vi "TTA_MATLAB_RFIC_Perform1TilePALTest.vi"(0 "Channel":string(combo), 1 "MXG VISA Resource In":refnum<visa-resource-name>, 2 "EXA VISA Resource":refnum<visa-resource-name>, 5 "Tx":string(combo), 7 "Freq_Cal_List":dbl[](array[numeric]), 11 "error in":errorcluster) -> (12 "MXG VISA Resource Out":refnum<visa-resource-name>, 13 "EXA VISA Resource Out":refnum<visa-resource-name>, 15 "error out":errorcluster)   [LabVIEW 2016]
uses:
  TTA_Globals/TTA_Global_Complete_Settings.vi
panel:
  out "IF Index":i32
  in  "PALLinearization Values":T1
  out "Tx#":i32
  out "CH#":i32
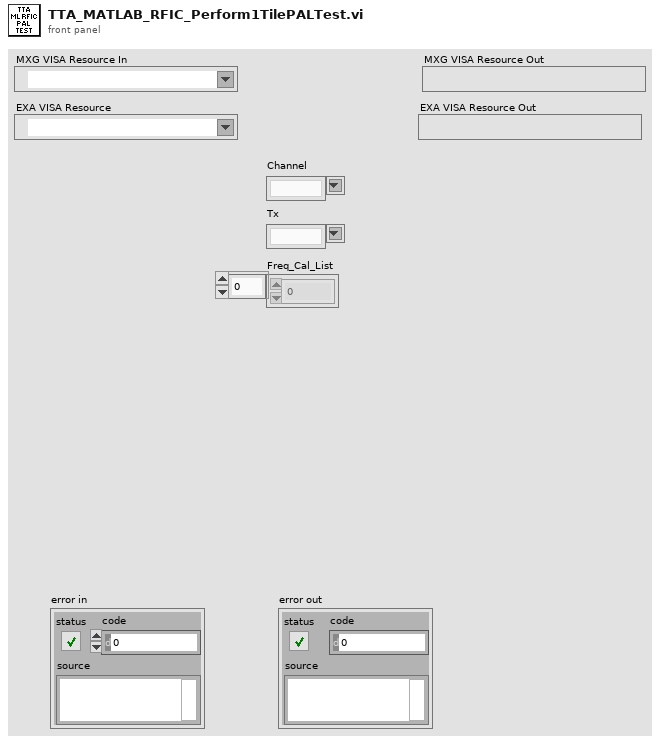
[diagram p1: front panel]
types:
  T1 = cluster{"Tx IF Offsets":dbl[], "ACPR Filename":string, "Sampling Rate":dbl, "TxIF_Freq":dbl, "Power (dBm)":dbl, "IF Frequency Sweep (MHz)":dbl[], "BDSFreq":dbl, "Amplitude Range\nMax(dBm)":dbl, "Amplitude Range\nMin(dBm)":dbl, "CAL Amplitude\nIncrement(dB)":dbl, "CAL Amplitude\nDecrement (dB)":dbl, "Amplitude Least\nCriteria (dBm)":dbl}
  T2 = typedef "TTA_Control_Complete_Settings_Cluster.ctl" = cluster{"Brief Cluster":cluster{"STM Firmware File":string, "STM Firmware Address":string, "Required SW Version":string, "Template Used":string}, "Instrument Setting Cluster":cluster{"BDSFreq":dbl, "BDS Amp":dbl, "TxRFCal_Freq":dbl, "TxRFCal_Amp":dbl, "RxRFCal_Freq":dbl, "RxRFCal_Freq":dbl, "TxIF_Freq":dbl, "TxIF_Amp":dbl, "Tx_Output_Power_Signal_Freq":dbl, "Tx_ACPR_Signal_Freq":dbl, "Rx_RF_Freq":dbl, "Rx_RF_Amp":dbl, "Rx_Output_Power_Signal_Freq":dbl, "Rx_Output_Power_Sense_Freq":dbl}, "PAL Calibration\nInputs Cluster":cluster{"Amplitude Range\nMax(dBm)":dbl, "Amplitude Range\nMin(dBm)":dbl, "Amplitude Least\nCriteria (dBm)":dbl, "Frequency 1":dbl, "Frequency 2":dbl, "Frequency 3":dbl, "CAL Amplitude\nDecrement (dB)":dbl, "CAL Amplitude\nIncrement(dB)":dbl, "DownloadFile":string}, "TxOffset Cal Cluster":cluster{"Tx1 Offset (dB)":dbl, "Tx2 Offset (dB)":dbl, "Tx3 Offset (dB)":dbl, "Tx4 Offset (dB)":dbl, "Total RF Tx Loss (dB)":dbl}, "RxOffset Cal Cluster":cluster{"Rx1 Offset (dB)":dbl, "Rx2 Offset (dB)":dbl, "Rx3 Offset (dB)":dbl, "Rx4 Offset (dB)":dbl, "Total RF Rx Loss (dB)":dbl}, "TX Output Power Settings Cluster":cluster{"Frequency Sweep (MHz)":dbl[], "Sig Gen \nPower (dBm)":dbl, "Span (kHz)":dbl, "RBW (Hz)":dbl, "Ref Level (dBm)":dbl, "Low Power \nLimit":dbl, "High Power \nLimit":dbl, "DigAtt Max":dbl, "DigAtt Min":dbl}, "Tx ACPR Settings Cluster":cluster{"ACPR Filename":string, "Sampling Rate":dbl, "Power (dBm)":dbl, "IF Frequency Sweep (MHz)":dbl[], "State Name":string, "Mechanical\nAttenuation":dbl, "RefLevel Offset":dbl, "Amplitude Range\nMax (dBm)":dbl, "Amplitude Range\nMin (dBm)":dbl, "Cal Amp \nIncrement (dB)":dbl, "Cal Amp\nDecrement (dB)":dbl}, "Power Cal Cluster":cluster{"Power List (dBm)":dbl[], "Frequency (MHz)":dbl[], "Cal Decrement (dB)":dbl, "Cal Increment (dB)":dbl}, "Rx Received Power Settings Cluster":cluster{"Frequency Sweep (MHz)":dbl[], "Power (dBm)":dbl, "Span (kHz)":dbl, "RBW (Hz)":dbl, "Ref Level":dbl, "Low Power \nLimit (dBm)":dbl, "High Power\nLimit (dBm)":dbl}, "Tx Output Power Criteria Cluster":cluster{"CH1-TX1 \nMin":dbl, "CH1-TX1\nMax":dbl, "CH1-TXx3\nMin ":dbl, "CH1-TXx3\nMax":dbl, "CH2-TX1\nMin":dbl, "CH2-TX1\nMax":dbl, "CH2-TXx3\nMin":dbl, "CH2-TXx3\nMax":dbl}, "Tx ACPR Criteria Cluster":cluster{"Min Inband":dbl, "Max Close Outband":dbl, "Max Far Outband":dbl}, "Rx Output Power Criteria Cluster":cluster{"CH1-RX1 \nMin":dbl, "CH1-RX1 \nMax":dbl, "CH1-RXx3 \nMin":dbl, "CH1-RXx3\nMax":dbl, "CH2-RX1\nMin":dbl, "CH2-RX1\nMax":dbl, "CH2-RXx3\nMin":dbl, "CH2-RXx3\nMax":dbl}}
  T3 = cluster{"BDSFreq":dbl, "BDS Amp":dbl, "TxRFCal_Freq":dbl, "TxRFCal_Amp":dbl, "RxRFCal_Freq":dbl, "RxRFCal_Freq":dbl, "TxIF_Freq":dbl, "TxIF_Amp":dbl, "Tx_Output_Power_Signal_Freq":dbl, "Tx_ACPR_Signal_Freq":dbl, "Rx_RF_Freq":dbl, "Rx_RF_Amp":dbl, "Rx_Output_Power_Signal_Freq":dbl, "Rx_Output_Power_Sense_Freq":dbl}
  T4 = cluster{"Amplitude Range\nMax(dBm)":dbl, "Amplitude Range\nMin(dBm)":dbl, "Amplitude Least\nCriteria (dBm)":dbl, "Frequency 1":dbl, "Frequency 2":dbl, "Frequency 3":dbl, "CAL Amplitude\nDecrement (dB)":dbl, "CAL Amplitude\nIncrement(dB)":dbl, "DownloadFile":string}
  T5 = cluster{"Tx1 Offset (dB)":dbl, "Tx2 Offset (dB)":dbl, "Tx3 Offset (dB)":dbl, "Tx4 Offset (dB)":dbl, "Total RF Tx Loss (dB)":dbl}
  T6 = cluster{"ACPR Filename":string, "Sampling Rate":dbl, "Power (dBm)":dbl, "IF Frequency Sweep (MHz)":dbl[], "State Name":string, "Mechanical\nAttenuation":dbl, "RefLevel Offset":dbl, "Amplitude Range\nMax (dBm)":dbl, "Amplitude Range\nMin (dBm)":dbl, "Cal Amp \nIncrement (dB)":dbl, "Cal Amp\nDecrement (dB)":dbl}
  T7 = cluster{"Amplitude Range\nMax(dBm)":dbl, "Amplitude Range\nMin(dBm)":dbl, "CAL Amplitude\nDecrement (dB)":dbl, "CAL Amplitude\nIncrement(dB)":dbl, "Amplitude Least\nCriteria (dBm)":dbl}
  T8 = enum16{"TX1", "TX2", "TX3", "TX4", "TXx3", "TXx4", "RX1", "RX2", "RX3", "RX4", "RXx3", "RXx4", "RFCal"}
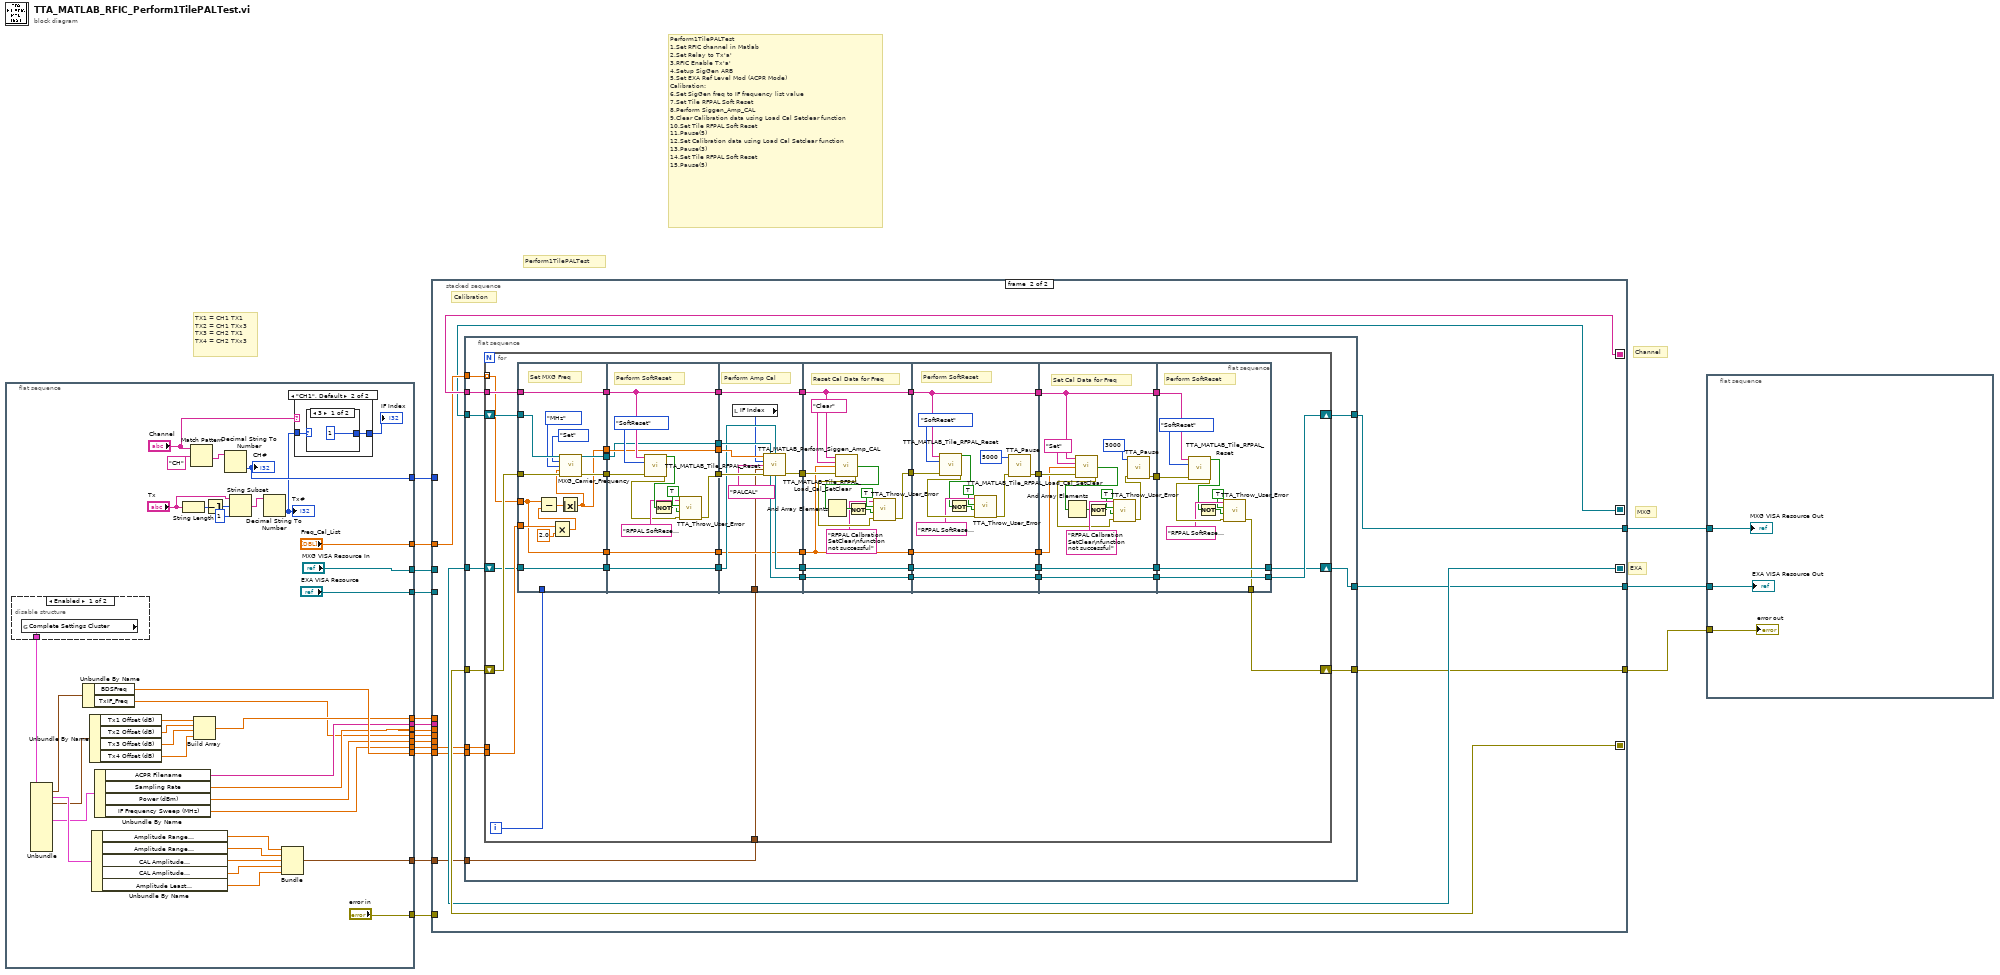
[diagram p0: block diagram]
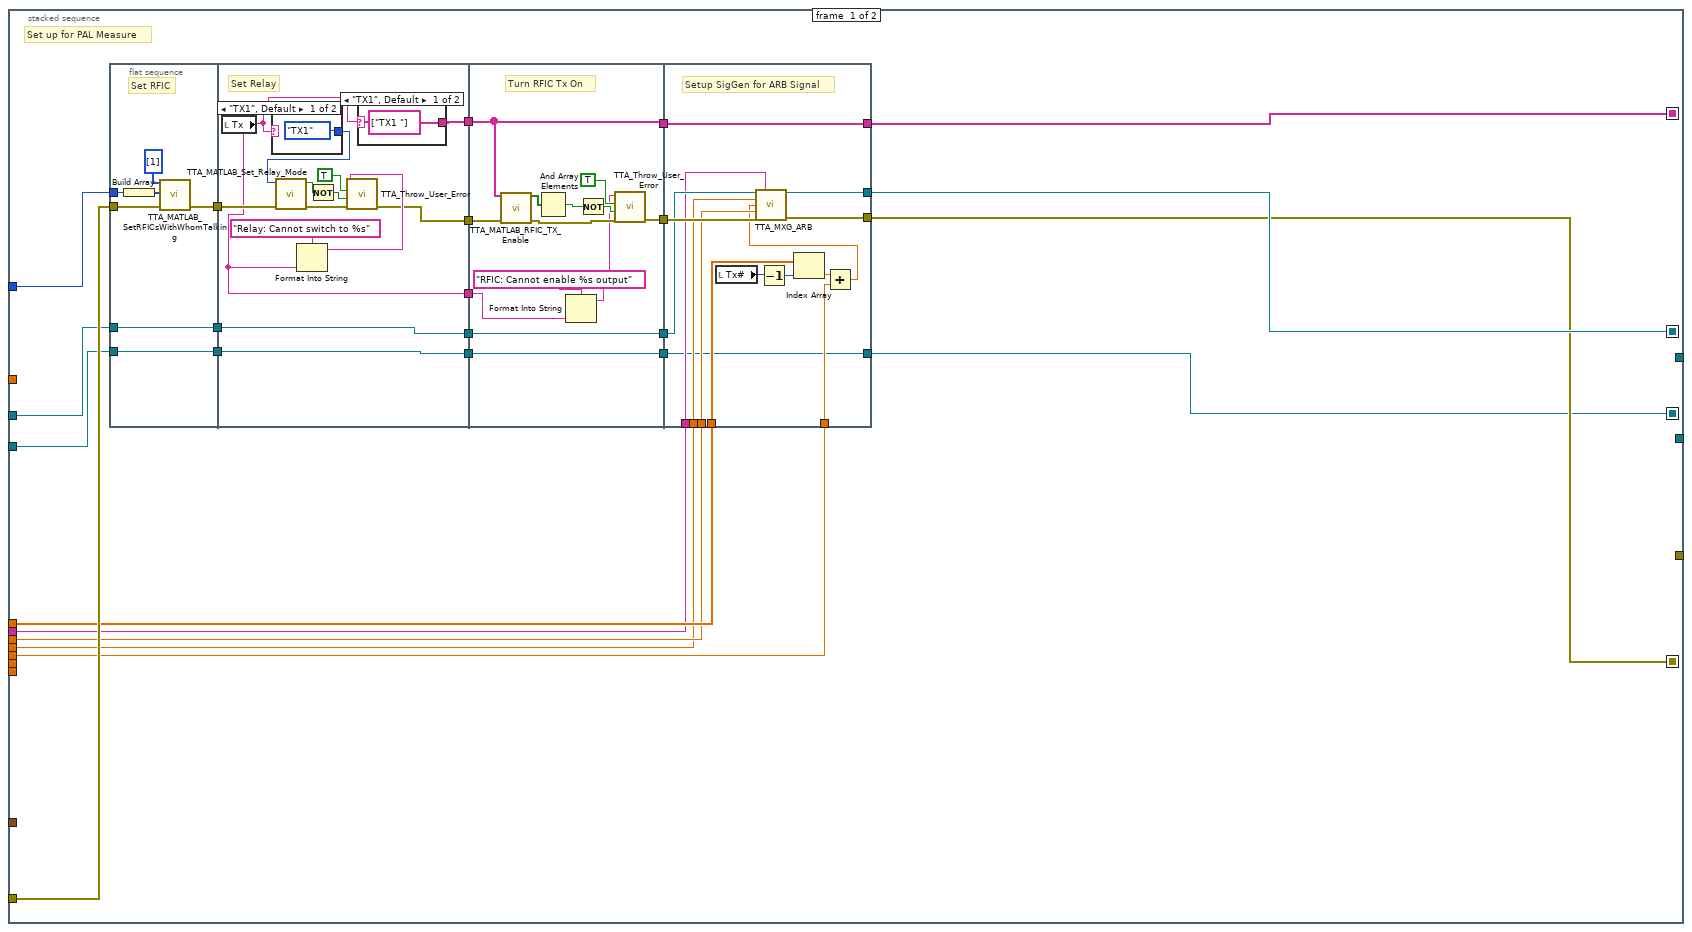
[diagram p2: hidden frame]
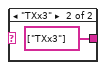
[diagram p3: hidden frame]
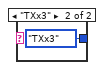
[diagram p4: hidden frame]
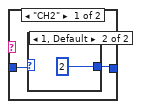
[diagram p5: hidden frame]
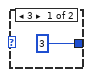
[diagram p6: hidden frame]
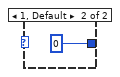
[diagram p7: hidden frame]
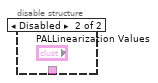
[diagram p8: hidden frame]
diagram:
  # "TX1 = CH1 TX1\nTX2 = CH1 TXx3\nTX3 = CH2 TX1\nTX4 = CH2 TXx3"
  # "Perform1TilePALTest\n1.Set RFIC channel in Matlab\n2.Set Relay to Tx'a'\n3.RFIC Enable Tx'a'\n4.Setup SigGen ARB\n5.Set EXA Ref Level Mod (ACPR Mode)\nCalibration:\n6.Set SigGen freq to IF frequency list value\n7.Set Tile RFPAL Soft Reset\n8.Perform Siggen_Amp_CAL \n9.Clear Calibration data using Load Cal Setclear function\n10.Set Tile RFPAL Soft Reset\n11.Pause(5)\n12.Set Calibration data using Load Cal Setclear function\n13.Pause(3)\n14.Set Tile RFPAL Soft Reset\n15.Pause(5)"
  # "EXA"
  # "MXG"
  # "Channel"
  # "Perform1TilePALTest"
  n1 = flat-sequence {
    tunnel: ["error in"] -> w16
    tunnel: ["MXG VISA Resource In"] -> w14
    tunnel: ["EXA VISA Resource"] -> w13
    tunnel: [w48] -> w15
    tunnel: ["Freq_Cal_List"] -> w10
    tunnel: [w27] -> w9
    tunnel: [w32] -> w8
    tunnel: [w30] -> w7
    tunnel: [w31] -> w6
    tunnel: [w29] -> w5
    tunnel: [w28] -> w4
    tunnel: [w37] -> w3
    tunnel: [w17] -> w2
    frame #0 {
      n2 = disable-structure shown="Enabled" {
        disable-tunnel: [w62 _] -> w42
        frame Enabled {
          n3 = global read "TTA_Global_Complete_Settings.vi" "Complete Settings Cluster"() -> (w62:T2)
        }
        frame Disabled {
        }
      }
      n4 = Unbundle(w42) -> ("Instrument Setting Cluster"=w41:T3, "PAL Calibration\nInputs Cluster"=w40:T4, "TxOffset Cal Cluster"=w39:T5, "Tx ACPR Settings Cluster"=w38:T6)  [unwired: 8 out]
      n5 = Unbundle By Name(w41) -> ("BDSFreq"=w37:dbl, "TxIF_Freq"=w27:dbl)
      n6 = Unbundle By Name(w39) -> ("Tx1 Offset (dB)"=w36:dbl, "Tx2 Offset (dB)"=w35:dbl, "Tx3 Offset (dB)"=w34:dbl, "Tx4 Offset (dB)"=w33:dbl)
      n7 = Unbundle By Name(w40) -> ("Amplitude Range\nMax(dBm)"=w22:dbl, "Amplitude Range\nMin(dBm)"=w21:dbl, "CAL Amplitude\nDecrement (dB)"=w20:dbl, "CAL Amplitude\nIncrement(dB)"=w19:dbl, "Amplitude Least\nCriteria (dBm)"=w18:dbl)
      n8 = Unbundle By Name(w38) -> ("ACPR Filename"=w31:string, "Sampling Rate"=w30:dbl, "Power (dBm)"=w29:dbl, "IF Frequency Sweep (MHz)"=w28:dbl[])
      n9 = String Length(string="Tx") -> (length=w47:i32)
      n10 = Match Pattern(string="Channel", regular expression="CH") -> (after substring=w49:string)  [unwired: 1 in, 3 out]
      n11 = Build Array(w36, w35, w34, w33) -> (w32:dbl[])
      n12 = Decrement(x=w47) -> (x-1=w46:i32)
      n13 = Decimal String To Number(string=w49) -> (number=w48:i32)  [unwired: 2 in, 1 out]
      "CH#" <- w48
      n14 = String Subset(string="Tx", offset (0)=w46, length (rest)=1 ("length (rest)")) -> (substring=w44:string)
      n15 = Decimal String To Number(string=w44) -> (number=w24:i32)  [unwired: 2 in, 1 out]
      "Tx#" <- w24
      n16 = Bundle("Amplitude Range\nMax(dBm)"=w22, "Amplitude Range\nMin(dBm)"=w21, "CAL Amplitude\nDecrement (dB)"=w20, "CAL Amplitude\nIncrement(dB)"=w19, "Amplitude Least\nCriteria (dBm)"=w18) -> (w17:T7)  [unwired: 1 in]
      n17 = case shown="\"CH1\", Default" "Channel" {
        tunnel: w24 -> [w54 w59]
        tunnel: [w55 w58] -> w23
        frame "CH2" {
          n18 = case shown="1, Default" w54 {
            tunnel: [3 2] -> w55
            frame 3 {
            }
            frame 1, Default {
            }
          }
        }
        frame "CH1", Default {
          n19 = case shown="3" w59 {
            tunnel: [1 0] -> w58
            frame 3 {
            }
            frame 1, Default {
            }
          }
        }
      }
      "IF Index" <- w23
    }
  }
  n20 = stacked-sequence {
    seq-local: [w64 _] -> [_ w150]
    seq-local: [w77 _] -> [_ w144]
    seq-local: [w63 _] -> [_ w148]
    seq-local: [w65 _] -> [_ w149]
    tunnel: w16 -> [w87 _]
    tunnel: w15 -> [w86 _]
    tunnel: w14 -> [w84 _]
    tunnel: w13 -> [w83 _]
    tunnel: [_ w143] -> w12
    tunnel: [_ w142] -> w11
    tunnel: w10 -> [_ w145]
    tunnel: w9 -> [w67 _]
    tunnel: w8 -> [w75 _]
    tunnel: w7 -> [w74 _]
    tunnel: w6 -> [w73 _]
    tunnel: w5 -> [w66 _]
    tunnel: w4 -> [_ w147]
    tunnel: w3 -> [_ w146]
    tunnel: w2 -> [_ w141]
    tunnel: [_ w140] -> w1
    frame #0 {
      # "Set up for PAL Measure"
      n21 = flat-sequence {
        tunnel: w87 -> [w94]
        tunnel: w86 -> [w91]
        tunnel: [w90] -> w85
        tunnel: w84 -> [w89]
        tunnel: w83 -> [w88]
        tunnel: [w89] -> w82
        tunnel: [w88] -> w81
        tunnel: w85 -> [w107]
        tunnel: w82 -> [w99]
        tunnel: w81 -> [w96]
        tunnel: [w99] -> w72
        tunnel: [w98] -> w71
        tunnel: [w97] -> w70
        tunnel: [w96] -> w69
        tunnel: [w95] -> w68
        tunnel: [w117] -> w80
        tunnel: w72 -> [w116]
        tunnel: [w116] -> w79
        tunnel: [w113] -> w78
        tunnel: [w115] -> w76
        tunnel: w71 -> [w115]
        tunnel: w70 -> [w114]
        tunnel: w69 -> [w113]
        tunnel: w68 -> [w112]
        tunnel: w80 -> [w135]
        tunnel: w79 -> [w133]
        tunnel: w78 -> [w125]
        tunnel: w76 -> [w127]
        tunnel: w75 -> [w136]
        tunnel: w74 -> [w134]
        tunnel: w73 -> [w132]
        tunnel: w67 -> [w131]
        tunnel: w66 -> [w130]
        tunnel: [w128] -> w77
        tunnel: [w127] -> w65
        tunnel: [w126] -> w64
        tunnel: [w125] -> w63
        frame #0 {
          # "Set RFIC"
          n22 = Build Array(w91) -> (w92:i32[])
          n23 = call "TTA_MATLAB_SetRFICsWithWhomTalking.vi"("Panel Array"=i32[] [1], "RFIC Array"=w92, "error in"=w94) -> ("error out"=w90:errorcluster)  [unwired: 12 in]
        }
        frame #1 {
          # "Set Relay"
          n24 = local read "Tx"() -> (w95:string)
          n25 = case shown="\"TX1\", Default" w95 {
            tunnel: [T8."TX1" ("Mode") T8."TXx3" ("Mode")] -> w106
            frame "TX1", Default {
            }
            frame "TXx3" {
            }
          }
          n26 = call "TTA_MATLAB_Set_Relay_Mode.vi"("error in"=w107, "Mode"=w106) -> ("error out"=w105:errorcluster, "Success"=w104:bool)  [unwired: 8 in]
          n27 = Format Into String(format string="Relay: Cannot switch to %s", w95) -> (resulting string=w100:string)  [unwired: 2 in, 1 out]
          n28 = Not(x=w104) -> (.not. x?=w103:bool)
          n29 = call "TTA_Throw_User_Error.vi"("error in"=w105, "Error?"=w103, "Stop Execution on Fail"=TRUE, "Error Message"=w100) -> ("error out"=w97:errorcluster)  [unwired: 7 in]
          n30 = case shown="\"TX1\", Default" w95 {
            tunnel: [string[] ["TX1 "] ("Channels") string[] ["TXx3"] ("Channels")] -> w98
            frame "TX1", Default {
            }
            frame "TXx3" {
            }
          }
        }
        frame #2 {
          # "Turn RFIC Tx On"
          n31 = call "TTA_MATLAB_RFIC_TX_Enable.vi"("Channels"=w115, "error in"=w114) -> ("SuccessComm"=w124:bool[], "error out"=w120:errorcluster)  [unwired: 12 in]
          n32 = And Array Elements(Boolean array=w124) -> (logical AND=w121:bool)
          n33 = Format Into String(format string="RFIC: Cannot enable %s output", w112) -> (resulting string=w118:string)  [unwired: 2 in, 1 out]
          n34 = Not(x=w121) -> (.not. x?=w122:bool)
          n35 = call "TTA_Throw_User_Error.vi"("error in"=w120, "Error?"=w122, "Stop Execution on Fail"=TRUE, "Error Message"=w118) -> ("error out"=w117:errorcluster)  [unwired: 7 in]
        }
        frame #3 {
          # "Setup SigGen for ARB Signal"
          n36 = local read "Tx#"() -> (w139:i32)
          n37 = Decrement(x=w139) -> (x-1=w138:i32)
          n38 = Index Array(array=w136, index=w138) -> (element=w137:dbl)
          n39 = Add(x=w137, y=w130) -> (x+y=w129:dbl)
          n40 = call "TTA_MXG_ARB.vi"("VISA resource In"=w133, "Waveform File"=w132, "Frequency (MHz)"=w131, "Output Power\nLevel (dBm)"=w129, "ARB Sample Rate"=w134, "error in"=w135) -> ("VISA resource Out"=w128:refnum<visa-resource-name>, "error out"=w126:errorcluster)  [unwired: 8 in]
        }
      }
    }
    frame #1 {
      # "Calibration"
      n41 = flat-sequence {
        tunnel: w150 -> [w161]
        tunnel: w149 -> [w160]
        tunnel: w148 -> [w159]
        tunnel: [w158] -> w143
        tunnel: [w157] -> w142
        tunnel: w147 -> [w156]
        tunnel: w146 -> [w155]
        tunnel: w145 -> [w154]
        tunnel: w144 -> [w153]
        tunnel: w141 -> [w152]
        tunnel: [w151] -> w140
        frame #0 {
          n42 = for {
            shift-right: [w163] -> w157
            shift-left: w161 -> [w200]
            tunnel: w160 -> [w197]
            shift-right: [w164] -> w158
            shift-left: w159 -> [w190]
            tunnel: w156 -> [_]
            tunnel: w155 -> [w202]
            tunnel: w154 -> [w184] mode=indexing
            shift-right: [w165] -> w151
            shift-left: w153 -> [w201]
            tunnel: w152 -> [w162]
            i -> [w203]
            n43 = flat-sequence {
              tunnel: w184 -> [w204]
              tunnel: w203 -> [_]
              tunnel: w202 -> [w213]
              tunnel: w201 -> [w216]
              tunnel: w200 -> [w217]
              tunnel: [w209] -> w199
              tunnel: [w208] -> w198
              tunnel: w197 -> [w207]
              tunnel: [w207] -> w196
              tunnel: [w206] -> w192
              tunnel: w190 -> [w205]
              tunnel: [w205] -> w188
              tunnel: [w204] -> w182
              tunnel: w199 -> [w220]
              tunnel: w198 -> [w230]
              tunnel: w196 -> [w222]
              tunnel: [w223] -> w195
              tunnel: [w222] -> w194
              tunnel: [w221] -> w193
              tunnel: w192 -> [w221]
              tunnel: [w220] -> w191
              tunnel: [w219] -> w189
              tunnel: w188 -> [w219]
              tunnel: w182 -> [w218]
              tunnel: [w218] -> w180
              tunnel: w195 -> [w242]
              tunnel: w194 -> [w234]
              tunnel: w193 -> [w240]
              tunnel: w191 -> [w239]
              tunnel: w189 -> [w236]
              tunnel: [w238] -> w187
              tunnel: [w237] -> w186
              tunnel: [w235] -> w185
              tunnel: [w234] -> w183
              tunnel: [w233] -> w181
              tunnel: w180 -> [w233]
              tunnel: w162 -> [w231]
              tunnel: w187 -> [w245]
              tunnel: w186 -> [w246]
              tunnel: w185 -> [w255]
              tunnel: w183 -> [w244]
              tunnel: w181 -> [w243]
              tunnel: [w247] -> w179
              tunnel: [w246] -> w178
              tunnel: [w245] -> w177
              tunnel: [w244] -> w176
              tunnel: [w243] -> w170
              tunnel: w179 -> [w263]
              tunnel: w178 -> [w262]
              tunnel: w177 -> [w261]
              tunnel: w176 -> [w257]
              tunnel: [w262] -> w175
              tunnel: [w261] -> w174
              tunnel: [w259] -> w173
              tunnel: [w257] -> w172
              tunnel: [w256] -> w171
              tunnel: w170 -> [w256]
              tunnel: w175 -> [w272]
              tunnel: w174 -> [w271]
              tunnel: w173 -> [w277]
              tunnel: w172 -> [w270]
              tunnel: w171 -> [w276]
              tunnel: [w274] -> w169
              tunnel: [w272] -> w168
              tunnel: [w271] -> w167
              tunnel: [w270] -> w166
              tunnel: [w294] -> w165
              tunnel: [w295] -> w164
              tunnel: w169 -> [w286]
              tunnel: w168 -> [w295]
              tunnel: w167 -> [w294]
              tunnel: w166 -> [w287]
              tunnel: [w285] -> w163
              frame #0 {
                # "Set MXG Freq"
                n44 = Multiply(x=w213, y=2.0) -> (x*y=w211:dbl)
                n45 = Subtract(x=w204, y=w211) -> (x-y=w210:dbl)
                n46 = Absolute Value(x=w210) -> (abs(x)=w206:dbl)
                n47 = call "MXG_Carrier_Frequency.vi"("VISA resource name"=w216, "Mode"=enum16{"Set", "Get"}."Set", "Units"=enum16{"Hz", "kHz", "MHz", "GHz"}."MHz", "Frequency"=w206, "error in"=w217) -> ("VISA resource name"=w209:refnum<visa-resource-name>, "error out"=w208:errorcluster)  [unwired: 8 in, 1 out]
              }
              frame #1 {
                # "Perform SoftReset"
                n48 = call "TTA_MATLAB_Tile_RFPAL_Reset.vi"("Channels"=w222, "Mode"=enum16{"SoftReset", "HardReset"}."SoftReset", "error in"=w230) -> ("Success"=w226:bool, "error out"=w224:errorcluster)  [unwired: 9 in, 2 out]
                n49 = Not(x=w226) -> (.not. x?=w227:bool)
                n50 = call "TTA_Throw_User_Error.vi"("error in"=w224, "Error?"=w227, "Stop Execution on Fail"=TRUE, "Error Message"="RFPAL SoftReset not successful") -> ("error out"=w223:errorcluster)  [unwired: 7 in]
              }
              frame #2 {
                # "Perform Amp Cal"
                n51 = local read "IF Index"() -> (w232:i32)
                n52 = call "TTA_MATLAB_Perform_Siggen_Amp_CAL.vi"("IF Frequency (MHz)"=w240, "MXG VISA Resource In"=w239, "EXA VISA Resource"=w236, "IF Index"=w232, "Test"="PALCAL", "Amp CAL Criteria Cluster"=w231, "error in"=w242) -> ("MXG VISA Resource Out"=w238:refnum<visa-resource-name>, "EXA VISA Resource Out"=w237:refnum<visa-resource-name>, "error out"=w235:errorcluster)  [unwired: 4 in, 2 out]
              }
              frame #3 {
                # "Reset Cal Data for Freq"
                n53 = call "TTA_MATLAB_Tile_RFPAL_Load_Cal_SetClear.vi"("Channels"=w244, "Mode"="Clear", "Frequency"=w243, "error in"=w255) -> ("TileSuccessComm"=w250:bool[], "error out"=w249:errorcluster)  [unwired: 8 in, 2 out]
                n54 = And Array Elements(Boolean array=w250) -> (logical AND=w251:bool)
                n55 = Not(x=w251) -> (.not. x?=w253:bool)
                n56 = call "TTA_Throw_User_Error.vi"("error in"=w249, "Error?"=w253, "Stop Execution on Fail"=TRUE, "Error Message"="RFPAL Calbration SetClear\nfunction not successful") -> ("error out"=w247:errorcluster)  [unwired: 7 in]
              }
              frame #4 {
                # "Perform SoftReset"
                n57 = call "TTA_MATLAB_Tile_RFPAL_Reset.vi"("Channels"=w257, "Mode"=enum16{"SoftReset", "HardReset"}."SoftReset", "error in"=w263) -> ("Success"=w267:bool, "error out"=w269:errorcluster)  [unwired: 9 in, 2 out]
                n58 = Not(x=w267) -> (.not. x?=w266:bool)
                n59 = call "TTA_Throw_User_Error.vi"("error in"=w269, "Error?"=w266, "Stop Execution on Fail"=TRUE, "Error Message"="RFPAL SoftReset not successful") -> ("error out"=w260:errorcluster)  [unwired: 7 in]
                n60 = call "TTA_Pause.vi"("error in"=w260, "Pause (ms)"=u32 5000) -> ("error out"=w259:errorcluster)  [unwired: 9 in]
              }
              frame #5 {
                # "Set Cal Data for Freq"
                n61 = call "TTA_MATLAB_Tile_RFPAL_Load_Cal_SetClear.vi"("Channels"=w270, "Mode"="Set", "Frequency"=w276, "error in"=w277) -> ("TileSuccessComm"=w282:bool[], "error out"=w283:errorcluster)  [unwired: 8 in, 2 out]
                n62 = And Array Elements(Boolean array=w282) -> (logical AND=w281:bool)
                n63 = Not(x=w281) -> (.not. x?=w279:bool)
                n64 = call "TTA_Throw_User_Error.vi"("error in"=w283, "Error?"=w279, "Stop Execution on Fail"=TRUE, "Error Message"="RFPAL Calbration SetClear\nfunction not successful") -> ("error out"=w275:errorcluster)  [unwired: 7 in]
                n65 = call "TTA_Pause.vi"("error in"=w275, "Pause (ms)"=u32 3000) -> ("error out"=w274:errorcluster)  [unwired: 9 in]
              }
              frame #6 {
                # "Perform SoftReset"
                n66 = call "TTA_MATLAB_Tile_RFPAL_Reset.vi"("Channels"=w287, "Mode"=enum16{"SoftReset", "HardReset"}."SoftReset", "error in"=w286) -> ("Success"=w291:bool, "error out"=w293:errorcluster)  [unwired: 9 in, 2 out]
                n67 = Not(x=w291) -> (.not. x?=w290:bool)
                n68 = call "TTA_Throw_User_Error.vi"("error in"=w293, "Error?"=w290, "Stop Execution on Fail"=TRUE, "Error Message"="RFPAL SoftReset not successful") -> ("error out"=w285:errorcluster)  [unwired: 7 in]
              }
            }
          }
        }
      }
    }
  }
  n69 = flat-sequence {
    tunnel: w12 -> [w298]
    tunnel: w11 -> [w297]
    tunnel: w1 -> [w296]
    frame #0 {
      "error out" <- w297
      "MXG VISA Resource Out" <- w296
      "EXA VISA Resource Out" <- w298
    }
  }
